vi "Globals.vi"() -> ()   [LabVIEW 2017]
panel:
  in  "IPv4 Message Counter":i16
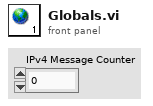
[diagram p1: front panel]
diagram:
